vi "Generate Unique Header.vi"(8 "error in (no error)":errorcluster, 11 "M data in":refnum<class "M data.lvclass">) -> (0 "error out":errorcluster, 2 "Header":string[](array[string]), 3 "M data out":refnum<class "M data.lvclass">)   [LabVIEW 2015, in "Alicat Lib.lvlib" / "M data.lvclass"]
uses:
  M data.lvclass
  Alicat Data.lvclass/Alicat Data.ctl
  Alicat Data.lvclass
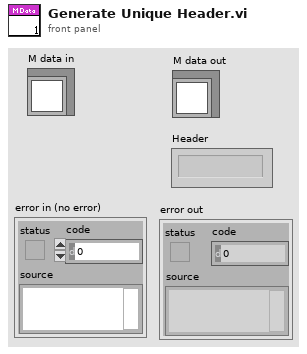
[diagram p1: front panel]
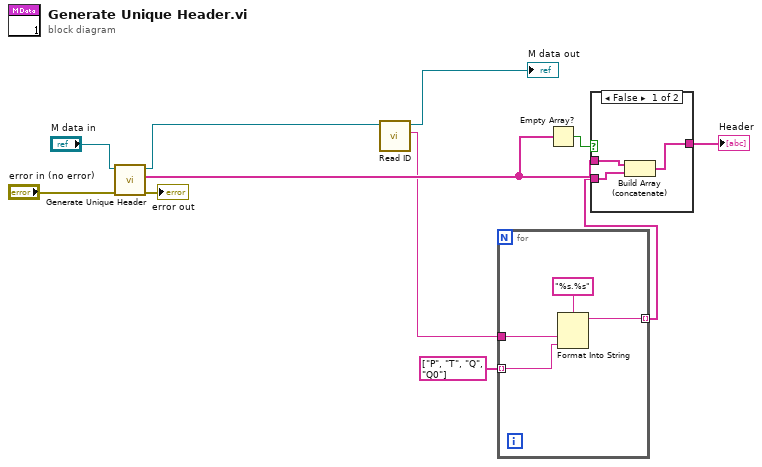
[diagram p0: block diagram]
diagram:
  n1 = call-parent "Generate Unique Header.vi"("error in"="error in (no error)", "Alicat Data in"="M data in") -> ("error out"=→"error out":errorcluster, "Header"=w4:string[], "Alicat Data out"=w6:refnum<class "M data.lvclass">)  [unwired: 7 in]
  n2 = call "Read ID.vi"("Alicat Data in"=w6) -> ("ID"=w2:string, "Alicat Data out"=→"M data out":refnum<class "M data.lvclass">)  [unwired: 8 in, 1 out]
  n3 = for {
    tunnel: string[] ["P", "T", "Q", "Q0"] -> [w13] mode=indexing
    tunnel: w2 -> [w14]
    tunnel: [w12] -> w1 mode=indexing
    n4 = Format Into String(format string="%s.%s", w14, w13) -> (resulting string=w12:string)  [unwired: 2 in, 1 out]
  }
  n5 = Empty Array?(array=w4) -> (empty?=w8:bool)
  n6 = case shown="False" w8 {
    tunnel: w1 -> [w18 w19]
    tunnel: [w16 w19] -> w7
    tunnel: w4 -> [w17 _]
    frame False {
      n7 = Build Array (concatenate)(w17, w18) -> (w16:string[])
    }
    frame True {
    }
  }
  "Header" <- w7
